vi "Gate Apply.vi"(8 "error in (no error)":errorcluster, 9 "Waveform in":dbl[](array[numeric]), 10 "Sampling Rate (Hz)":dbl, 11 "Gate Control":T1(xcontrol)) -> (0 "error out":errorcluster, 1 "Gated waveform":dbl[](array[numeric]))   [LabVIEW 2020]
uses:
  Controls/Gate XCtl/Gate Control.xctl
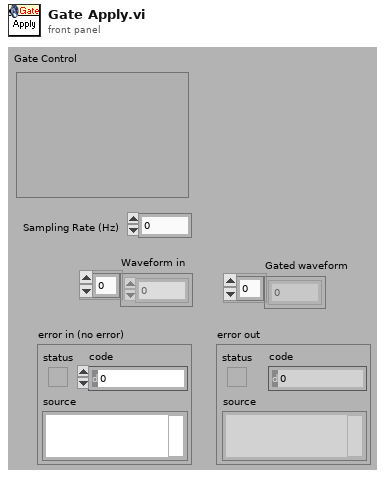
[diagram p1: front panel]
types:
  T1 = cluster{"Active":bool, "Delay (ms)":dbl, "Width (ms)":dbl, "Ramp (ms)":dbl}
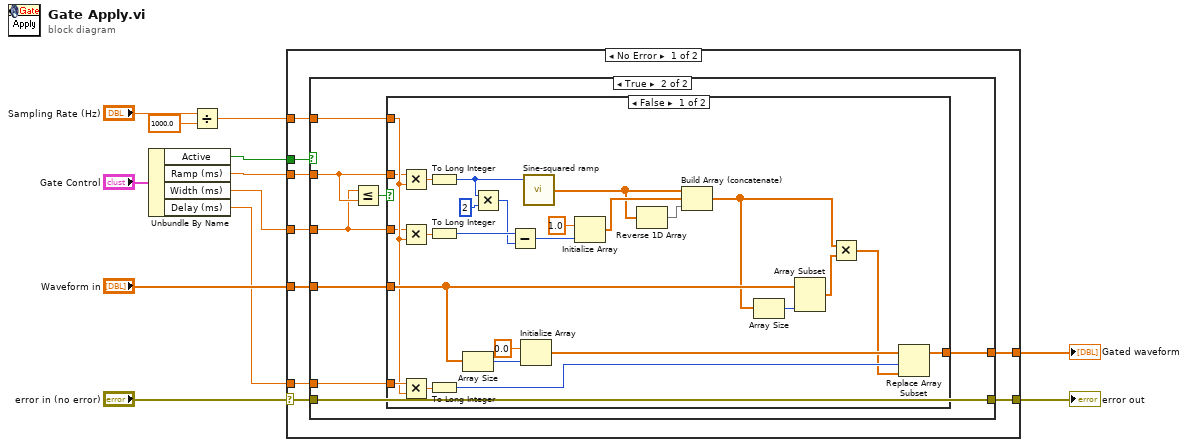
[diagram p0: block diagram]
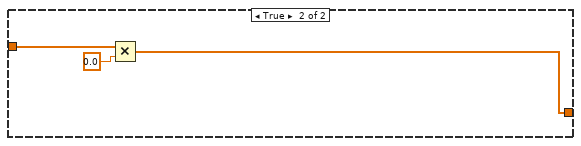
[diagram p3: hidden frame]
diagram:
  n1 = Unbundle By Name("Gate Control") -> ("Active"=w10:bool, "Ramp (ms)"=w6:dbl, "Width (ms)"=w2:dbl, "Delay (ms)"=w1:dbl)
  n2 = Divide(x="Sampling Rate (Hz)", y=1000.0) -> (x/y=w3:dbl)
  n3 = case shown="No Error" "error in (no error)" {
    selector: "error in (no error)" -> [w14 w61]
    tunnel: w10 -> [w21 _]
    tunnel: "Waveform in" -> [w20 _]
    tunnel: [w19 _] -> w8
    tunnel: [w13 w61] -> w7
    tunnel: w6 -> [w18 _]
    tunnel: w3 -> [w17 _]
    tunnel: w2 -> [w16 _]
    tunnel: w1 -> [w15 _]
    frame No Error {
      n4 = case shown="True" w21 {
        tunnel: w20 -> [w23 w31]
        tunnel: [w23 w28] -> w19
        tunnel: w18 -> [_ w26]
        tunnel: w17 -> [_ w29]
        tunnel: w16 -> [_ w25]
        tunnel: w15 -> [_ w30]
        tunnel: w14 -> [w22 w27]
        tunnel: [w22 w27] -> w13
        frame False {
        }
        frame True {
          n5 = Less Or Equal?(x=w25, y=w26) -> (x <= y?=w24:bool)
          n6 = case shown="False" w24 {
            tunnel: w31 -> [w43 w60]
            tunnel: w30 -> [w41 _]
            tunnel: w29 -> [w40 _]
            tunnel: [w36 w58] -> w28
            tunnel: w26 -> [w35 _]
            tunnel: w25 -> [w34 _]
            frame False {
              n7 = Multiply(x=w35, y=w40) -> (x*y=w57:dbl)
              n8 = Multiply(x=w34, y=w40) -> (x*y=w54:dbl)
              n9 = Multiply(x=w41, y=w40) -> (x*y=w42:dbl)
              n10 = To Long Integer(number=w57) -> (32bit integer=w56:i32)
              n11 = To Long Integer(number=w54) -> (32bit integer=w53:i32)
              n12 = To Long Integer(number=w42) -> (32bit integer=w38:i32)
              n13 = Array Size(array=w43) -> (size(s)=w44:i32)
              n14 = Multiply(x=w56, y=2) -> (x*y=w52:i32)
              n15 = Subtract(x=w53, y=w52) -> (x-y=w51:i32)
              n16 = Initialize Array(0.0 ("element"), w44) -> (w39:dbl[])
              n17 = call "Sine-squared ramp.vi"("samples"=w56) -> ("sine^2 Ramp"=w32:dbl[])  [unwired: 3 in, 1 out]
              n18 = Initialize Array(1.0 ("element"), w51) -> (w49:dbl[])
              n19 = Reverse 1D Array(array=w32) -> (reversed array=w48:dbl[])
              n20 = Build Array (concatenate)(w32, w49, w48) -> (w33:dbl[])
              n21 = Array Size(array=w33) -> (size(s)=w47:i32)
              n22 = Array Subset(array=w43, length=w47) -> (w46:dbl[])  [unwired: 1 in]
              n23 = Multiply(x=w33, y=w46) -> (x*y=w37:dbl[])
              n24 = Replace Array Subset(array=w39, new element=w37, index=w38) -> (w36:dbl[])
            }
            frame True {
              n25 = Multiply(x=w60, y=0.0) -> (x*y=w58:dbl[])
            }
          }
        }
      }
    }
    frame Error {
    }
  }
  "error out" <- w7
  "Gated waveform" <- w8
